vi "WriteRead Data.vi"(5 "Address":T1 format="%02x", 6 "NoStop (F)":bool, 7 "I2C":refnum<class "I2C.lvclass">, 8 "error in (no error)":errorcluster, 9 "Len":u8, 10 "Write Data":string, 11 "Session In":refnum<class "Session.lvclass">) -> (0 "error out":errorcluster, 1 "Read Data":string, 3 "Session Out":refnum<class "Session.lvclass">)   [LabVIEW 2020, in "CTI.lvlib" / "I2C.lvclass"]
uses:
  I2C.lvclass
  I2C.lvclass/I2C.ctl
  Session/Session.lvclass
  I2C Address.ctl
  CTI.lvlib
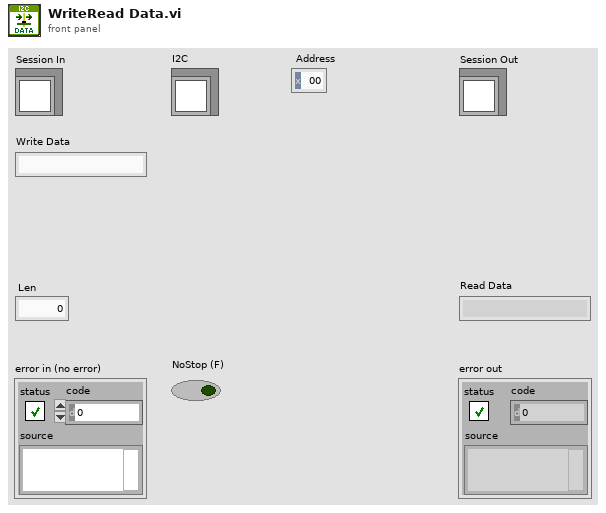
[diagram p1: front panel]
types:
  T1 = typedef "CTI.lvlib/I2C Address.ctl" = u8
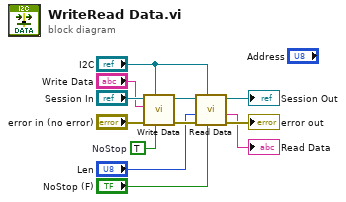
[diagram p0: block diagram]
diagram:
  w9 = TRUE  # NoStop
  n1 = call "Write Data.vi"("NoStop (F)"=w9, "I2C"="I2C", "error in (no error)"="error in (no error)", "Data"="Write Data", "Session In"="Session In") -> ("error out"=w8:errorcluster, "Session Out"=w7:refnum<class "Session.lvclass">)  [unwired: 5 in]
  n2 = call "Read Data.vi"("NoStop (F)"="NoStop (F)", "I2C"="I2C", "error in (no error)"=w8, "Len"="Len", "Session In"=w7) -> ("error out"=→"error out":errorcluster, "Data"=→"Read Data":string, "Session Out"=→"Session Out":refnum<class "Session.lvclass">)  [unwired: 4 in]
